vi "1.vi"() -> ()   [LabVIEW 2022 SP3]
panel:
  out "Volume":dbl(slide) scale=0.0..10.0
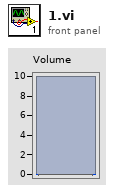
[diagram p1: front panel]
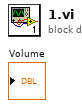
[diagram p0: block diagram]
diagram:
